vi "Config Type.vi"(11 "Numeric Command in":refnum<class "Numeric Command.lvclass">) -> (2 "Command Config Type":refnum<class "Command Config.lvclass">)   [LabVIEW 2020, in "VolatusSeq.lvlib" / "Numeric Command.lvclass"]
uses:
  Numeric Command.lvclass
  Numeric Command.lvclass/Numeric Command.ctl
  VolatusSeqConfig/Numeric Command Config/Numeric Command Config.lvclass
  C:/dev/lv20CE/relink/lv-volatus/VolatusSeqConfig/Command Config/Command Config.lvclass
  C:/dev/lv20CE/relink/lv-volatus/VolatusSeqConfig/Numeric Command Config/Numeric Command Config.lvclass
  VolatusSeqConfig/Command Config/Command Config.lvclass
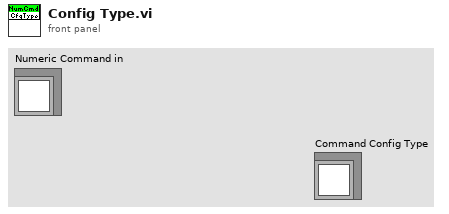
[diagram p1: front panel]
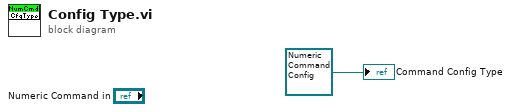
[diagram p0: block diagram]
diagram:
  "Command Config Type" <- refnum<class "Numeric Command Config.lvclass"> refnum ("VolatusSeqConfig.lvlib:Numeric Command Config.lvclass")
